vi "MotionProfiles_GetStatus.vi"(0 "MotionProfiles in":refnum<class "MotionProfiles.lvclass">, 11 "error in (no error)":errorcluster) -> (4 "MotionProfiles out":refnum<class "MotionProfiles.lvclass">, 8 "MP_Class_Status":T1, 15 "error out":errorcluster)   [LabVIEW 2018, in "MotionProfiles.lvclass"]
uses:
  MotionProfiles.lvclass
  MotionProfile_MP_Class_Status.ctl
  MotionProfile_TalonSetValueEnum.ctl
  MotionProfiles.lvclass/MotionProfiles.ctl
  <vilib>/Rock Robotics/WPI/ThirdParty/Phoenix-LabVIEW/Motor Controller/Get/CTRE_Phoenix_MotorController_GetVoltage.vi
  <vilib>/Rock Robotics/WPI/ThirdParty/Phoenix-LabVIEW/Motor Controller/Get/CTRE_Phoenix_MotorController_GetSelectedSensorData.vi
panel:
  in  "MP_Class_Status 2":T1
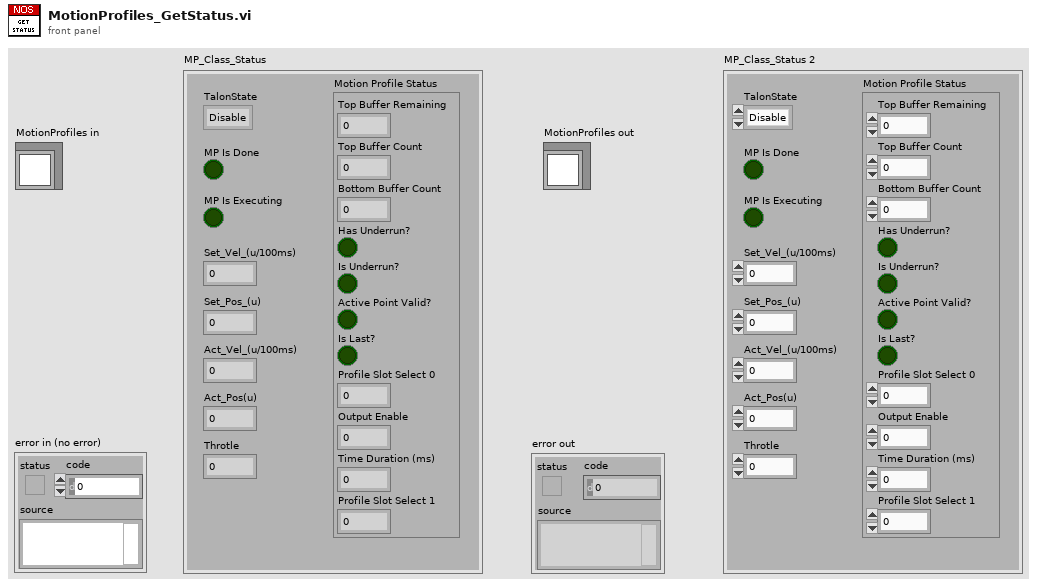
[diagram p1: front panel]
types:
  T1 = typedef "MotionProfiles.lvclass/MotionProfile_MP_Class_Status.ctl" = cluster{"Motion Profile Status":cluster{"Top Buffer Remaining":i32, "Top Buffer Count":i32, "Bottom Buffer Count":i32, "Has Underrun?":bool, "Is Underrun?":bool, "Active Point Valid?":bool, "Is Last?":bool, "Profile Slot Select 0":i32, "Output Enable":i32, "Time Duration (ms)":i32, "Profile Slot Select 1":i32}, "TalonState":T2, "MP Is Done":bool, "MP Is Executing":bool, "Set_Vel_(u/100ms)":i32, "Set_Pos_(u)":i32, "Act_Vel_(u/100ms)":i32, "Act_Pos(u)":i32, "Throtle":dbl}
  T2 = typedef "MotionProfiles.lvclass/MotionProfile_TalonSetValueEnum.ctl" = enum16{"Disable", "Enable", "Hold"}
  T3 = cluster{"Top Buffer Remaining":i32, "Top Buffer Count":i32, "Bottom Buffer Count":i32, "Has Underrun?":bool, "Is Underrun?":bool, "Active Point Valid?":bool, "Is Last?":bool, "Profile Slot Select 0":i32, "Output Enable":i32, "Time Duration (ms)":i32, "Profile Slot Select 1":i32}
  T4 = typedef "WPI_MotorControlDeviceRef.ctl" = cluster{"DeviceStatus":errorcluster, "Type":T5, "PWM":cluster{"PWM Channel":T6, "DeadBand":T7}, "CAN":cluster{"Device Number":u8, "SetOutput VI Ref":variant, "GetOutput VI Ref":variant, "Enable VI Ref":variant, "Disable VI Ref":variant, "Data":variant}, "Invert":bool, "DIO PWM":cluster{"PWM \"Enable\" Channel":T6, "DIOChannel":T8, "PWM Rate":dbl}}
  T5 = typedef "WPI_MotorControlType.ctl" = enum16{"PWM", "CAN", "DIO PWM"}
  T6 = typedef "FPGA_DIOPWMChannel.ctl" = enum8{"PWM 0", "PWM 1", "PWM 2", "PWM 3", "PWM 4", "PWM 5", "PWM 6", "PWM 7", "PWM 8", "PWM 9", "PWM MXP 0", "PWM MXP 1", "PWM MXP 2", "PWM MXP 3", "PWM MXP 4", "PWM MXP 5", "PWM MXP 6", "PWM MXP 7", "PWM MXP 8", "PWM MXP 9", "Invalid"}
  T7 = typedef "WPI_PWMDeadband.ctl" = cluster{"Name":string, "maxPositivePwm":i32, "minPositivePwm":i32, "centerPwm":i32, "maxNegativePwm":i32, "minNegativePwm":i32, "angularRange":u16}
  T8 = typedef "FPGA_DIOChannel.ctl" = enum8{"DIO 0", "DIO 1", "DIO 2", "DIO 3", "DIO 4", "DIO 5", "DIO 6", "DIO 7", "DIO 8", "DIO 9", "DIO MXP 0", "DIO MXP 1", "DIO MXP 2", "DIO MXP 3", "DIO MXP 4", "DIO MXP 5", "DIO MXP 6", "DIO MXP 7", "DIO MXP 8", "DIO MXP 9", "DIO MXP 10", "DIO MXP 11", "DIO MXP 12", "DIO MXP 13", "DIO MXP 14", "DIO MXP 15", "SPI Port CS1", "SPI Port CS2", "SPI Port CS3", "SPI Port MISO", "SPI Port MOSI", "Invalid"}
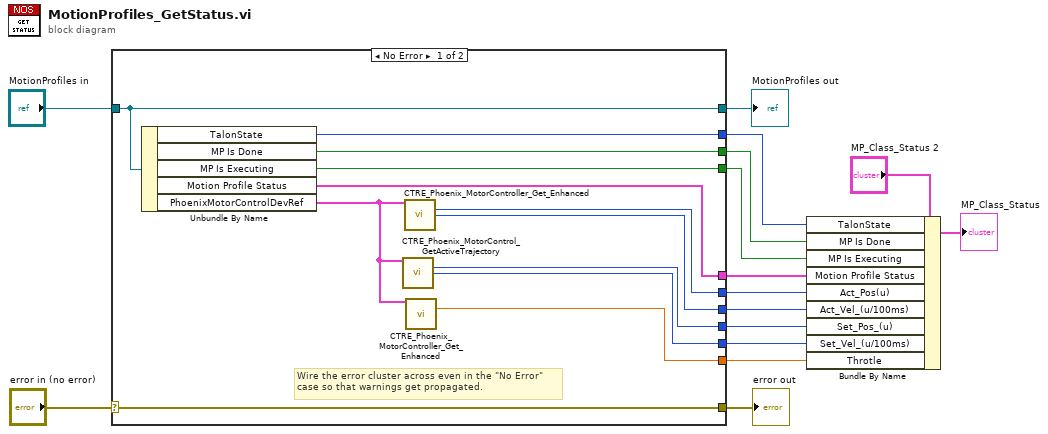
[diagram p0: block diagram]
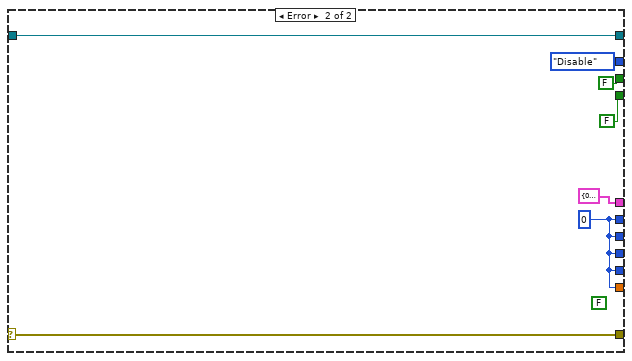
[diagram p2: hidden frame]
diagram:
  n1 = case shown="No Error" "error in (no error)" {
    selector: "error in (no error)" -> [w27 w34]
    tunnel: [w27 w34] -> w14
    tunnel: [w26 w33] -> w12
    tunnel: "MotionProfiles in" -> [w26 w33]
    tunnel: [w25 MotionProfile_TalonSetValueEnum."Disable" ("TalonSetValue")] -> w7
    tunnel: [w24 FALSE ("MP Is Done")] -> w8
    tunnel: [w23 T3 {"Top Buffer Remaining"=0, "Top Buffer Count"=0, "Bottom Buffer Count"=0, "Has Underrun?"=FALSE, "Is Underrun?"=FALSE, "Active Point Valid?"=FALSE, "Is Last?"=FALSE, "Profile Slot Select 0"=0, "Output Enable"=0, "Time Duration (ms)"=0, "Profile Slot Select 1"=0} ("Motion Profile Status")] -> w9
    tunnel: [w22 FALSE ("MP Is Executing")] -> w11
    tunnel: [w21 w28] -> w5
    tunnel: [w20 w28] -> w4
    tunnel: [w19 w28] -> w3
    tunnel: [w18 w28] -> w2
    tunnel: [w16 w28] -> w1
    frame No Error {
      # "Wire the error cluster across even in the \"No Error\"\ncase so that warnings get propagated."
      n2 = Unbundle By Name(w26) -> ("TalonState"=w25:T2, "MP Is Done"=w24:bool, "MP Is Executing"=w22:bool, "Motion Profile Status"=w23:T3, "PhoenixMotorControlDevRef"=w17:T4)
      n3 = call <vilib>:"CTRE_Phoenix_MotorControl_GetActiveTrajectory.vi"("PhoenixMotorControlDevRef"=w17) -> ("Position (Sensor Units)"=w19:i32, "Velocity (Sensor Units per 100 ms)"=w18:i32)  [unwired: 10 in, 3 out]
      n4 = call-poly <vilib>:"CTRE_Phoenix_MotorController_Get_Enhanced.vi"("PhoenixMotorControlDevRef"=w17) -> ("Position (Raw Sensor Units)"=w21:i32, "Velocity (Raw Sensor Units per 100 ms)"=w20:i32)  [unwired: 11 in, 2 out]
      n5 = call-poly <vilib>:"CTRE_Phoenix_MotorController_Get_Enhanced.vi"("PhoenixMotorControlDevRef"=w17) -> ("Percent Output"=w16:dbl)  [unwired: 10 in, 4 out]
    }
    frame Error {
      (unwired) FALSE ("Is Inverted?")
      w28 = 0 ("Position (Raw Sensor Units)")
    }
  }
  "error out" <- w14
  "MotionProfiles out" <- w12
  n6 = Bundle By Name(cluster="MP_Class_Status 2", "TalonState"=w7, "MP Is Done"=w8, "MP Is Executing"=w11, "Motion Profile Status"=w9, "Act_Pos(u)"=w5, "Act_Vel_(u/100ms)"=w4, "Set_Pos_(u)"=w3, "Set_Vel_(u/100ms)"=w2, "Throtle"=w1) -> (→"MP_Class_Status":T1)
